vi "Collate_graphs.vi"(4 "R values":dbl[](array[numeric]), 5 "rho0":dbl[](array[numeric]), 6 "rho-":dbl[](array[numeric]), 7 "rho+":dbl[](array[numeric]), 8 "Gaussian SD in":dbl, 9 "AFP Range":cluster{"Numeric":i32, "Numeric 2":i32}, 10 "RF Range 2":cluster{"Numeric":i32, "Numeric 2":i32}, 11 "RF Range 1":cluster{"Numeric":i32, "Numeric 2":i32}) -> (0 "Q_total out":dbl, 1 "P_total out":dbl, 2 "Q Graph":cluster{"Array":dbl[], "Array 2":dbl[]}, 3 "P Graph and Intensities and RF":cluster{"Array":dbl[], "Array":dbl[]}[](array[cluster]))   [LabVIEW 2018]
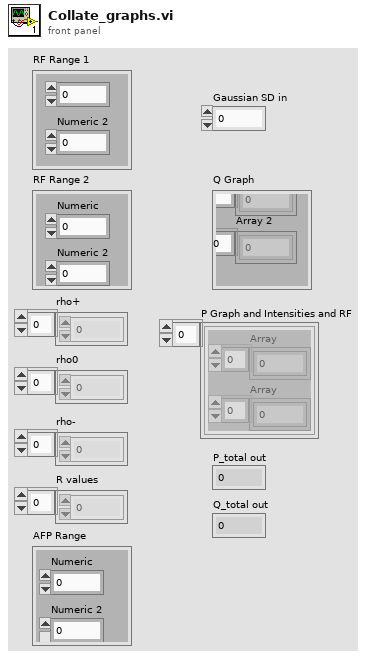
[diagram p1: front panel]
types:
  T1 = cluster{"R values":dbl[], "Output Array":dbl[]}[]
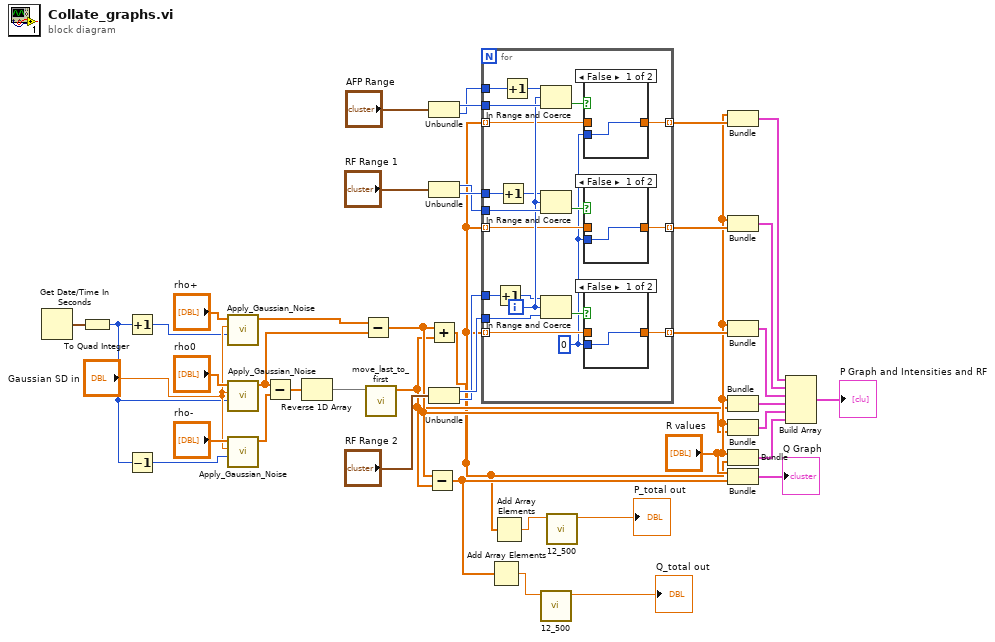
[diagram p0: block diagram]
diagram:
  n1 = Get Date/Time In Seconds() -> (seconds since 1Jan1904=w10:timestamp)
  n2 = To Quad Integer(1:w10) -> (0:w7:i64)
  n3 = Increment(x=w7) -> (x+1=w8:i64)
  n4 = Decrement(x=w7) -> (x-1=w9:i64)
  n5 = call "Apply_Gaussian_Noise.vi"("Seed in"=w8, "Gaussian SD in"="Gaussian SD in", "Array in"="rho+") -> ("Array out"=w14:dbl[])  [unwired: 8 in]
  n6 = call "Apply_Gaussian_Noise.vi"("Seed in"=w7, "Gaussian SD in"="Gaussian SD in", "Array in"="rho0") -> ("Array out"=w13:dbl[])  [unwired: 8 in]
  n7 = call "Apply_Gaussian_Noise.vi"("Seed in"=w9, "Gaussian SD in"="Gaussian SD in", "Array in"="rho-") -> ("Array out"=w12:dbl[])  [unwired: 8 in]
  n8 = Subtract(x=w13, y=w12) -> (x-y=w39:dbl[])
  n9 = Reverse 1D Array(array=w39) -> (reversed array=w16:dbl[])
  n10 = Subtract(x=w14, y=w13) -> (x-y=w19:dbl[])
  n11 = call "move_last_to_first.vi"("Input array"=w16) -> ("Output Array"=w15:dbl[])  [unwired: 10 in]
  n12 = Subtract(x=w19, y=w15) -> (x-y=w6:dbl[])
  n13 = Unbundle("AFP Range") -> ("Numeric"=w31:i32, "Numeric 2"=w30:i32)
  n14 = Unbundle("RF Range 1") -> ("Numeric"=w34:i32, "Numeric 2"=w35:i32)
  n15 = Add(x=w19, y=w15) -> (x+y=w5:dbl[])
  n16 = Unbundle("RF Range 2") -> ("Numeric"=w33:i32, "Numeric 2"=w32:i32)
  n17 = for {
    tunnel: w35 -> [w62]
    tunnel: w34 -> [w61]
    tunnel: w33 -> [w57]
    tunnel: w32 -> [w56]
    tunnel: w31 -> [w55]
    tunnel: w30 -> [w54]
    tunnel: w5 -> [w52] mode=indexing
    tunnel: w5 -> [w51] mode=indexing
    tunnel: w5 -> [w50] mode=indexing
    tunnel: [w49] -> w29 mode=indexing
    tunnel: [w48] -> w27 mode=indexing
    tunnel: [w47] -> w28 mode=indexing
    i -> [w53]
    w46 = 0
    n18 = Increment(x=w56) -> (x+1=w45:i32)
    n19 = Increment(x=w62) -> (x+1=w44:i32)
    n20 = Increment(x=w54) -> (x+1=w43:i32)
    n21 = In Range and Coerce(upper limit=w43, x=w53, lower limit=w55) -> (In Range?=w60:bool)  [unwired: 1 out]
    n22 = In Range and Coerce(upper limit=w44, x=w53, lower limit=w61) -> (In Range?=w58:bool)  [unwired: 1 out]
    n23 = In Range and Coerce(upper limit=w45, x=w53, lower limit=w57) -> (In Range?=w59:bool)  [unwired: 1 out]
    n24 = case shown="False" w60 {
      tunnel: w50 -> [_ w64]
      tunnel: [w63 w64] -> w47
      tunnel: w46 -> [w63 _]
      frame False {
      }
      frame True {
      }
    }
    n25 = case shown="False" w58 {
      tunnel: w52 -> [_ w68]
      tunnel: [w67 w68] -> w49
      tunnel: w46 -> [w67 _]
      frame False {
      }
      frame True {
      }
    }
    n26 = case shown="False" w59 {
      tunnel: w51 -> [_ w66]
      tunnel: [w65 w66] -> w48
      tunnel: w46 -> [w65 _]
      frame False {
      }
      frame True {
      }
    }
  }
  n27 = Add Array Elements(numeric array=w6) -> (sum=w4:dbl)
  n28 = Add Array Elements(numeric array=w5) -> (sum=w3:dbl)
  n29 = call "12_500.vi"("Numeric in"=w4) -> ("Numeric out"=→"Q_total out":dbl)  [unwired: 10 in]
  n30 = call "12_500.vi"("Numeric in"=w3) -> ("Numeric out"=→"P_total out":dbl)  [unwired: 10 in]
  n31 = Bundle("R values"="R values", w28) -> (w22:cluster{"R values":dbl[], dbl[]})  [unwired: 1 in]
  n32 = Bundle("R values"="R values", w29) -> (w26:cluster{"R values":dbl[], dbl[]})  [unwired: 1 in]
  n33 = Bundle("R values"="R values", w27) -> (w25:cluster{"R values":dbl[], dbl[]})  [unwired: 1 in]
  n34 = Bundle("R values"="R values", "Output Array"=w15) -> (w17:cluster{"R values":dbl[], "Output Array":dbl[]})  [unwired: 1 in]
  n35 = Bundle("R values"="R values", w19) -> (w18:cluster{"R values":dbl[], dbl[]})  [unwired: 1 in]
  n36 = Bundle("R values"="R values", w5) -> (w21:cluster{"R values":dbl[], dbl[]})  [unwired: 1 in]
  n37 = Bundle("R values"="R values", w6) -> (→"Q Graph":cluster{"R values":dbl[], dbl[]})  [unwired: 1 in]
  n38 = Build Array(w22, w26, w25, w17, w18, w21) -> (→"P Graph and Intensities and RF":T1)
